vi "Sets_Union(TimeStamp).vi"(8 "error in (no error)":errorcluster caption="错误输入（无错误）", 10 "输入数组B":timestamp[](array[timestamp]), 11 "输入数组A":timestamp[](array[timestamp])) -> (0 "error out":errorcluster caption="错误输出", 3 "输出数组C":timestamp[](array[timestamp]))   [LabVIEW 2012]
uses:
  Sets_Unique(TimeStamp).vi
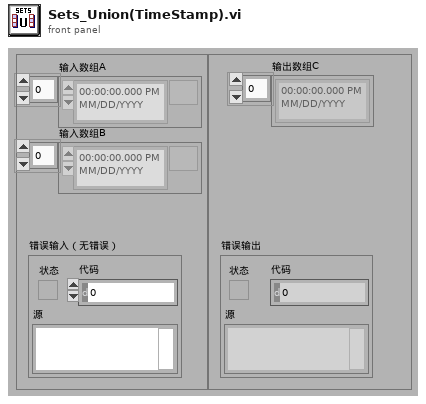
[diagram p1: front panel]
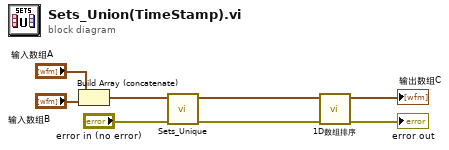
[diagram p0: block diagram]
diagram:
  n1 = Build Array (concatenate)("输入数组A", "输入数组B") -> (w4:timestamp[])
  n2 = call-poly "Sets_Unique.vi"("error in (no error)"="error in (no error)", "输入数组"=w4) -> ("error out"=w2:errorcluster, "输出数组"=w3:timestamp[])  [unwired: 7 in, 1 out]
  n3 = call-poly "1D数组排序.vi"("error in (no error)"=w2, "输入数组"=w3) -> ("error out"=→"error out":errorcluster, "排序后数组"=→"输出数组C":timestamp[])  [unwired: 7 in, 1 out]
